vi "myRIO v1.0 Reserve AudioIn Block.vi"(7 "Allow multiple opens?":bool, 8 "error in (no error)":errorcluster, 10 "AudioIn (N Samples) Channel List":T2, 11 "Generic FPGA Reference":T1) -> (0 "error out":errorcluster)   [LabVIEW 2021]
uses:
  <vilib>/myRIO/Common/Instrument Driver Framework/myRIO v1.0/AudioIn Block/typedefs/AudioIn Block Channels List.ctl
  <vilib>/myRIO/Common/Instrument Driver Framework/myRIO v1.0/AudioIn Block/typedefs/AudioIn Block Channels Enum.ctl
  <vilib>/myRIO/Common/Instrument Driver Framework/Utilities/typedefs/Generic FPGA Reference.ctl
  <vilib>/myRIO/Common/Instrument Driver Framework/myRIO v1.0/AudioIn Block/typedefs/AudioIn Block Channels FPGA Reference.ctl
  <vilib>/myRIO/Common/Instrument Driver Framework/myRIO v1.0/Resource Manager/vis/myRIO v1.0 Reserve Channel.vi
  <vilib>/myRIO/Common/Instrument Driver Framework/myRIO v1.0/Resource Manager/vis/myRIO v1.0 Unreserve Channel.vi
  <vilib>/myRIO/Common/Instrument Driver Framework/myRIO v1.0/Resource Manager/vis/myRIO v1.0 Build Mutex Name.vi
  <vilib>/myRIO/Common/Instrument Driver Framework/myRIO v1.0/Resource Manager/vis/myRIO v1.0 Block Write Configuration.vi
  <vilib>/myRIO/Common/Instrument Driver Framework/Utilities/vis/IO Manager.vi
  <vilib>/Utility/error.llb/Error Cluster From Error Code.vi
  <vilib>/myRIO/Common/Instrument Driver Framework/Utilities/vis/Configuration Manager.vi
  <vilib>/rvi/interface/common/niFpgaWaitOnOcc.vi
  <vilib>/rvi/interface/nirviMethod/nirviMethod.xnode
  <vilib>/FPGAPlugInAG/Dynamic/niLvFpga_ConfigureFifo_Dynamic.vi
  <vilib>/rvi/errors/niLvFpgaMergeErrorWithErrorCode.vi
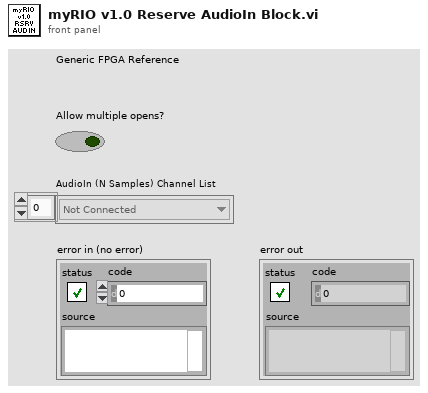
[diagram p1: front panel]
types:
  T1 = typedef "Generic FPGA Reference.ctl" = refnum<k20>
  T2 = typedef "AudioIn Block Channels List.ctl" = T3[]
  T3 = typedef "AudioIn Block Channels Enum.ctl" = enum16{"Not Connected", "AudioIn/Left (N Samples)", "AudioIn/Right (N Samples)"}
  T4 = typedef "AudioIn Block Channels FPGA Reference.ctl" = refnum<k20>
  T5 = typedef "myRIO v1.0 Channel Reservation List.ctl" = T6[]
  T6 = typedef "myRIO v1.0 Channel Reservation Info.ctl" = cluster{"Channel Name":string, "Connector":T7, "Mutex ID":i32}
  T7 = typedef "myRIO v1.0 Connector List.ctl" = enum32{"None", "ConnectorA", "ConnectorB", "ConnectorC"}
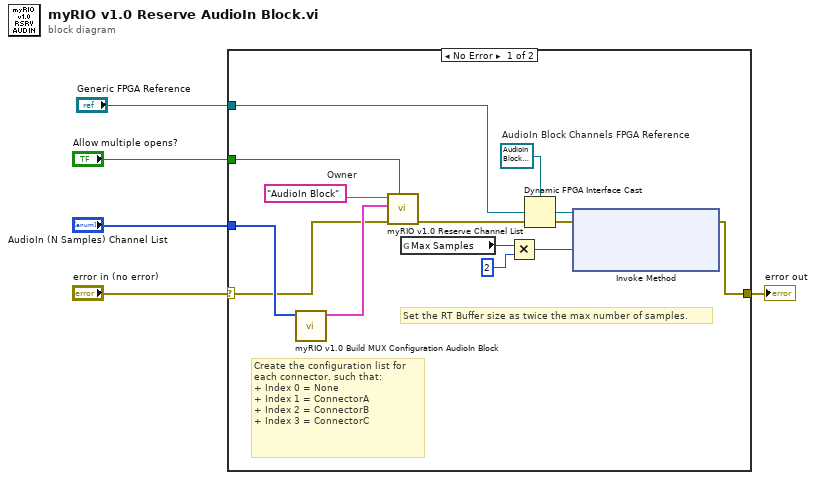
[diagram p0: block diagram]
diagram:
  n1 = case shown="No Error" "error in (no error)" {
    selector: "error in (no error)" -> [w15 w19]
    tunnel: "Allow multiple opens?" -> [w14 _]
    tunnel: "AudioIn (N Samples) Channel List" -> [w18 _]
    tunnel: [w6 w19] -> w4
    tunnel: "Generic FPGA Reference" -> [w13 _]
    frame No Error {
      w12 = T4 refnum  # AudioIn Block Channels FPGA Reference
      w17 = "AudioIn Block"  # Owner
      # "Create the configuration list for each connector. such that:\n+ Index 0 = None\n+ Index 1 = ConnectorA\n+ Index 2 = ConnectorB \n+ Index 3 = ConnectorC"
      # "Set the RT Buffer size as twice the max number of samples."
      n2 = call <vilib>:"myRIO v1.0 Build MUX Configuration AudioIn Block.vi"("AudioIn (N Samples) Channels List"=w18) -> ("Channel Reservation Info"=w16:T5)  [unwired: 10 in]
      n3 = call <vilib>:"myRIO v1.0 Reserve Channel List.vi"("Allow multiple opens?"=w14, "error in (no error)"=w15, "Channel Reservation List"=w16, "Owner"=w17) -> ("error out"=w7:errorcluster)  [unwired: 7 in]
      n4 = global read "myRIO v1.0 Block Write Configuration.vi" "Max Samples"() -> (w11:u32)
      n5 = Multiply(x=w11, y=u32 2) -> (x*y=w8:u32)
      n6 = Dynamic FPGA Interface Cast(Session In=w12, Type=w13) -> (Session Out=w9:T4)
      n7 = xnode "Invoke Method"("FPGA VI Reference In"=w9, "error in"=w7, "Requested Depth"=w8) -> ("error out"=w6:errorcluster)  [unwired: 2 out]
    }
    frame Error {
      # "There is an incoming error so there is nothing to do."
    }
  }
  "error out" <- w4
